vi "DriveGetYawModulo.vi"() -> (3 "YawModulo":dbl)   [LabVIEW 2023]
doc: "Put global variable Gyro Z into Yaw to use in other VI's\n\nOutputs:\n -- Yaw -- Double -- Yaw of robot (rotation) --"
uses:
  DriveGlobal.vi
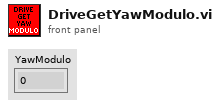
[diagram p1: front panel]
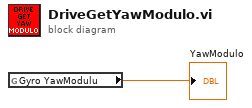
[diagram p0: block diagram]
diagram:
  n1 = global read "DriveGlobal.vi" "Gyro YawModulu"() -> (→"YawModulo":dbl)
